vi "Identify.vi"(8 "error in (no error)":errorcluster, 10 "Hello Msg":refnum<class "Hello.lvclass">, 11 "OBS in":refnum<class "OBS.lvclass">) -> (0 "error out":errorcluster, 2 "Identify Msg":refnum<class "Identify.lvclass">, 3 "OBS out":refnum<class "OBS.lvclass">)   [LabVIEW 2020, in "obs-websocket.lvlib" / "OBS.lvclass"]
uses:
  OBS.lvclass
  Hello/Hello.lvclass
  Identify/Identify.lvclass
  OBS.lvclass/OBS.ctl
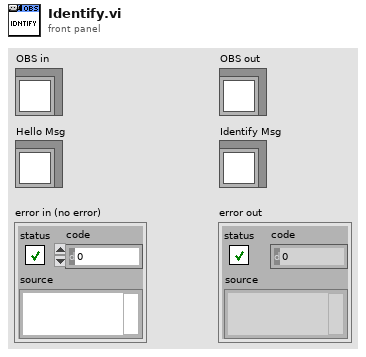
[diagram p1: front panel]
types:
  T1 = typedef "obs-websocket.lvlib/Authentication.ctl" = cluster{"Has Authentication":bool, "Salt":string, "Challenge":string}
  T2 = typedef "obs-websocket.lvlib/Event Subscription.ctl" = u32
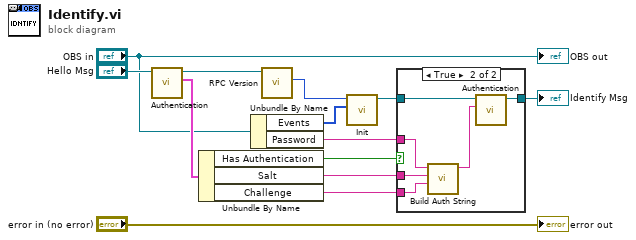
[diagram p0: block diagram]
diagram:
  n1 = call "Authentication.vi"("Hello in"="Hello Msg") -> ("Authentication"=w11:T1, "Hello out"=w4:refnum<class "Hello.lvclass">)  [unwired: 8 in, 1 out]
  n2 = Unbundle By Name(w11) -> ("Has Authentication"=w5:bool, "Salt"=w8:string, "Challenge"=w7:string)
  n3 = Unbundle By Name("OBS in") -> ("Events"=w1:T2[], "Password"=w9:string)
  n4 = call "RPC Version.vi"("Hello in"=w4) -> ("RPC Version"=w2:i32)  [unwired: 8 in, 2 out]
  n5 = call "Init.vi"("Event Subs (All)"=w1, "RPC Version"=w2) -> ("Identify out"=w3:refnum<class "Identify.lvclass">)  [unwired: 8 in, 1 out]
  n6 = case shown="True" w5 {
    tunnel: w9 -> [_ w20]
    tunnel: w8 -> [_ w19]
    tunnel: w7 -> [_ w18]
    tunnel: w3 -> [w14 w17]
    tunnel: [w14 w15] -> w6
    frame False {
    }
    frame True {
      n7 = call "Build Auth String.vi"("Challenge"=w18, "Salt"=w19, "Password"=w20) -> ("Auth String"=w16:string)  [unwired: 8 in]
      n8 = call "Authentication.vi"("Authentication"=w16, "Identify in"=w17) -> ("Identify out"=w15:refnum<class "Identify.lvclass">)  [unwired: 8 in, 1 out]
    }
  }
  "Identify Msg" <- w6
  "error out" <- "error in (no error)"
  "OBS out" <- "OBS in"
